vi "Contour Line_Find Candidate Edges (col).vi"(11 "edge":T2) -> (3 "Candidate Edges":T1(array[cluster]))   [LabVIEW 2020, in "NI_AAL_Geometry.lvlib"]
uses:
  <vilib>/Analysis/NI_AAL_Geometry.lvlib
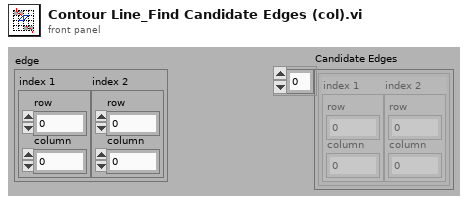
[diagram p1: front panel]
types:
  T1 = cluster{"index 1":cluster{"row":i32, "column":i32}, "index 2":cluster{"row":i32, "column":i32}}[]
  T2 = cluster{"index 1":cluster{"row":i32, "column":i32}, "index 2":cluster{"row":i32, "column":i32}}
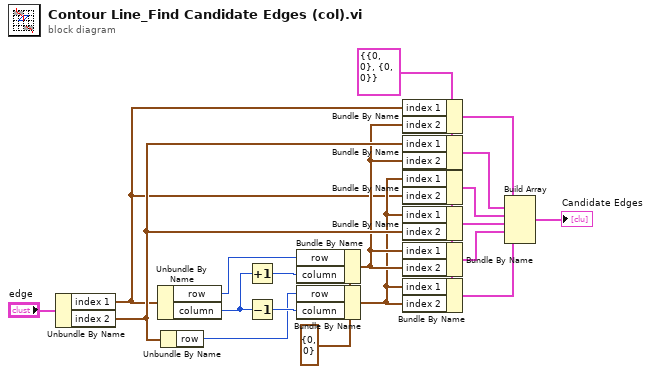
[diagram p0: block diagram]
diagram:
  w18 = cluster{"row":i32, "column":i32} {"row"=0, "column"=0} ("index 2")
  w17 = T2 {"index 1"={"row"=0, "column"=0}, "index 2"={"row"=0, "column"=0}} ("edge")
  n1 = Unbundle By Name("edge") -> ("index 1"=w1:cluster{"row":i32, "column":i32}, "index 2"=w4:cluster{"row":i32, "column":i32})
  n2 = Unbundle By Name(w1) -> ("row"=w8:i32, "column"=w7:i32)
  n3 = Unbundle By Name(w4) -> ("row"=w5:i32)
  n4 = Increment(x=w7) -> (x+1=w9:i32)
  n5 = Decrement(x=w7) -> (x-1=w6:i32)
  n6 = Bundle By Name(cluster=w18, "row"=w8, "column"=w9) -> (w3:cluster{"row":i32, "column":i32})
  n7 = Bundle By Name(cluster=w18, "row"=w5, "column"=w6) -> (w2:cluster{"row":i32, "column":i32})
  n8 = Bundle By Name(cluster=w17, "index 1"=w1, "index 2"=w3) -> (w16:T2)
  n9 = Bundle By Name(cluster=w17, "index 1"=w4, "index 2"=w3) -> (w15:T2)
  n10 = Bundle By Name(cluster=w17, "index 1"=w2, "index 2"=w1) -> (w14:T2)
  n11 = Bundle By Name(cluster=w17, "index 1"=w2, "index 2"=w4) -> (w13:T2)
  n12 = Bundle By Name(cluster=w17, "index 1"=w3, "index 2"=w3) -> (w12:T2)
  n13 = Bundle By Name(cluster=w17, "index 1"=w2, "index 2"=w2) -> (w11:T2)
  n14 = Build Array(w16, w15, w14, w13, w12, w11) -> (→"Candidate Edges":T1)
